vi "Set IPS PSU Target.vi"(6 "Axis":T1=enum."Z", 8 "error in (no error)":errorcluster, 9 "Target Field Rate (T/min)":dbl format="%#.2f", 10 "Target Field (T)":dbl format="%#.2f", 11 "Instrument.OxfordVRM in":refnum<class "Instrument.OxfordVRM.lvclass">) -> (0 "error out":errorcluster, 2 "Response":string, 3 "Instrument.OxfordVRM out":refnum<class "Instrument.OxfordVRM.lvclass">)   [LabVIEW 2019, in "Instrument.OxfordVRM.lvclass"]
uses:
  Instrument.OxfordVRM.lvclass
  <userlib>/LevyLab/Instrument Framework/Instrument Types/Cryostat/Typedefs/Magnet Axis--Enum.ctl
  Instrument.OxfordVRM.lvclass/Instrument.OxfordVRM.ctl
  <instrlib>/Mercury iXX/Public/Libraries/Magnet/Open/Open Magnet Device.vi
  <instrlib>/Mercury iXX/Public/Libraries/Magnet/Signals/Set/Target Field Rate (Set).vi
  <instrlib>/Mercury iXX/Public/Libraries/Magnet/Signals/Set/Target Field (Set).vi
  <instrlib>/Mercury iXX/Public/Libraries/Magnet/Signals/Read/Target Field Rate (Read).vi
  <instrlib>/Mercury iXX/Public/Libraries/Magnet/Signals/Read/Target Field (Read).vi
  <instrlib>/Mercury iXX/Mercury iXX.lvlib
  <instrlib>/Mercury iXX/Public/Libraries/Magnet.lvlib
  <userlib>/LevyLab/Instrument Framework/Instrument Types/Cryostat/Instrument.Cryostat.lvclass
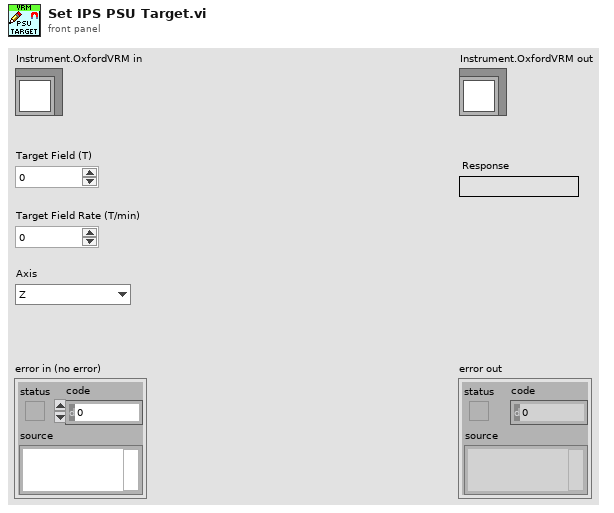
[diagram p1: front panel]
types:
  T1 = typedef "Instrument.Cryostat.lvclass/Magnet Axis--Enum.ctl" = enum16{"X", "Y", "Z"}
  T2 = typedef "Mercury iXX.lvlib/Mercury Reference.ctl" = cluster{"Comms":refnum<visa-resource-name>, "Device ID":string[], "Comms Layer":T3, "Command":string, "Query reference":T4}
  T3 = typedef "Mercury iXX.lvlib/Comms Transport Layer.ctl" = enum16{"Ethernet TCP/IP", "USB", "ISOBus - RS-232", "GPIB"}
  T4 = typedef "Mercury iXX.lvlib/Query Dynamic Reference.ctl" = refnum<vi>
  T5 = typedef "Mercury iXX.lvlib/Response String.ctl" = string
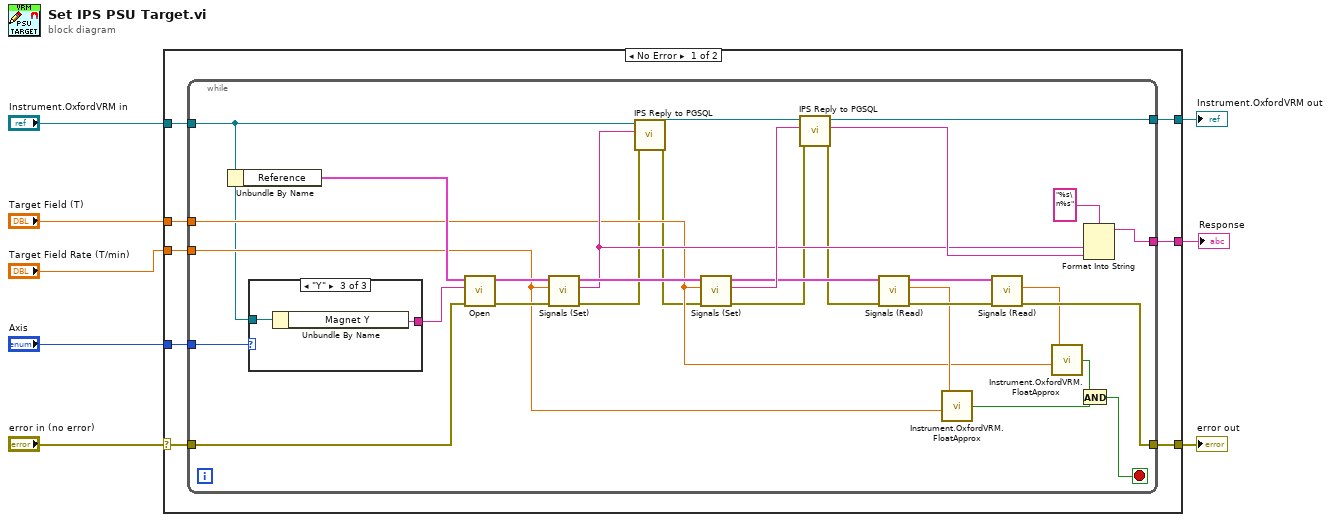
[diagram p0: block diagram]
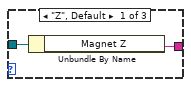
[diagram p2: hidden frame]
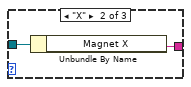
[diagram p3: hidden frame]
diagram:
  n1 = case shown="No Error" "error in (no error)" {
    selector: "error in (no error)" -> [w16 w53]
    tunnel: [w12 w53] -> w7
    tunnel: [w10 w52] -> w5
    tunnel: "Instrument.OxfordVRM in" -> [w9 w52]
    tunnel: [w13 _] -> w4
    tunnel: "Target Field (T)" -> [w15 _]
    tunnel: "Target Field Rate (T/min)" -> [w14 _]
    tunnel: "Axis" -> [w11 _]
    frame No Error {
      n2 = while {
        tunnel: w9 -> [w22]
        tunnel: w16 -> [w44]
        tunnel: w15 -> [w26]
        tunnel: w14 -> [w27]
        tunnel: [w37] -> w13
        tunnel: [w33] -> w12
        tunnel: w11 -> [w25]
        tunnel: [w21] -> w10
        stop <- w28 stop-if-true
        n3 = Unbundle By Name(w22) -> ("Reference"=w45:T2)
        n4 = case shown="\"Y\"" w25 {
          tunnel: [w47 w49 w50] -> w24
          tunnel: w22 -> [w46 w48 w51]
          frame "Z", Default {
            n5 = Unbundle By Name(w46) -> ("Magnet Z"=w47:string)
          }
          frame "X" {
            n6 = Unbundle By Name(w48) -> ("Magnet X"=w49:string)
          }
          frame "Y" {
            n7 = Unbundle By Name(w51) -> ("Magnet Y"=w50:string)
          }
        }
        n8 = call-poly <instrlib>:"Open.vi"("error in (no error)"=w44, "Device Identifier"=w24, "Mercury Reference In"=w45) -> ("error out"=w41:errorcluster, "Mercury Reference Out"=w42:T2)  [unwired: 7 out]
        n9 = call-poly <instrlib>:"Signals (Set).vi"("error in"=w41, "Target Field Rate"=w27, "Mercury Reference In"=w42) -> ("error out"=w18:errorcluster, "Response"=w38:T5, "Mercury Reference Out"=w43:T2)  [unwired: 2 in, 4 out]
        n10 = call "IPS Reply to PGSQL.vi"("error in (no error)"=w18, "Response"=w38, "Instrument.VRM in"=w22) -> ("error out"=w17:errorcluster, "Instrument.VRM out"=w23:refnum<class "Instrument.OxfordVRM.lvclass">)  [unwired: 7 in]
        n11 = call-poly <instrlib>:"Signals (Set).vi"("error in"=w17, "Target Field"=w26, "Mercury Reference In"=w43) -> ("error out"=w20:errorcluster, "Response"=w39:T5, "Mercury Reference Out"=w36:T2)  [unwired: 2 in, 4 out]
        n12 = call "IPS Reply to PGSQL.vi"("error in (no error)"=w20, "Response"=w39, "Instrument.VRM in"=w23) -> ("error out"=w19:errorcluster, "Instrument.VRM out"=w21:refnum<class "Instrument.OxfordVRM.lvclass">)  [unwired: 7 in]
        n13 = call-poly <instrlib>:"Signals (Read).vi"("error in"=w19, "Mercury Reference In"=w36) -> ("error out"=w34:errorcluster, "Target Field Rate"=w32:dbl, "Mercury Reference Out"=w35:T2)  [unwired: 5 in, 2 out]
        n14 = call "Instrument.OxfordVRM.FloatApprox.vi"("y"=w27, "x"=w32) -> ("x ~ y?"=w29:bool)  [unwired: 4 in]
        n15 = call-poly <instrlib>:"Signals (Read).vi"("error in"=w34, "Mercury Reference In"=w35) -> ("error out"=w33:errorcluster, "Target Field"=w31:dbl)  [unwired: 5 in, 3 out]
        n16 = call "Instrument.OxfordVRM.FloatApprox.vi"("y"=w26, "x"=w31) -> ("x ~ y?"=w30:bool)  [unwired: 4 in]
        n17 = And(x=w30, y=w29) -> (x .and. y?=w28:bool)
        n18 = Format Into String(format string="%s\n%s", w38, w39) -> (resulting string=w37:string)  [unwired: 2 in, 1 out]
      }
    }
    frame Error {
    }
  }
  "error out" <- w7
  "Instrument.OxfordVRM out" <- w5
  "Response" <- w4
